vi "setFIFO.vi"(0 "fifoThs":u8, 2 "fifoMode":u8) -> ()   [LabVIEW 2016]
uses:
  #defines.ctl
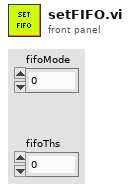
[diagram p1: front panel]
types:
  T1 = typedef "#defines.ctl" = i8
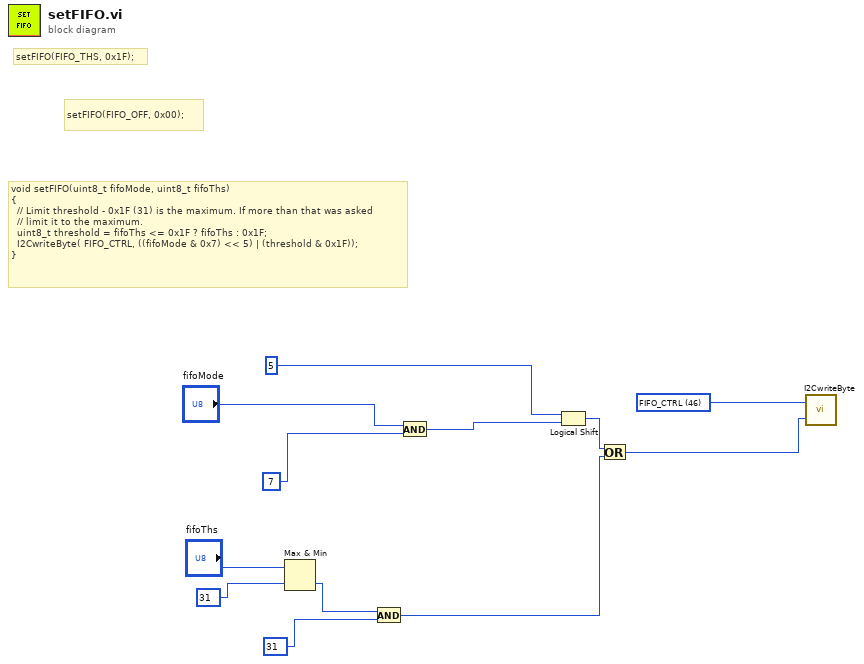
[diagram p0: block diagram]
diagram:
  w8 = T1 46 items=["CTRL_REG9_G"=35, "STATUS_REG_1"=39, "OUT_X_L_XL"=40, "FIFO_CTRL"=46, "FIFO_SRC"=47, "CTRL_REG4_G"=30, "OUT_X_L_G"=24, "OUT_TEMP_L"=21, "INT_GEN_SRC_G"=20, "ORIENT_CFG_G"=19, "CTRL_REG3_G"=18, "CTRL_REG2_G"=17, "CTRL_REG1_G"=16, "WHO_AM_I_XG"=15] ("Ring")
  # "setFIFO(FIFO_OFF, 0x00);"
  # "setFIFO(FIFO_THS, 0x1F);"
  # "void setFIFO(uint8_t fifoMode, uint8_t fifoThs)\n{\n  // Limit threshold - 0x1F (31) is the maximum. If more than that was asked\n  // limit it to the maximum.\n  uint8_t threshold = fifoThs <= 0x1F ? fifoThs : 0x1F;\n  I2CwriteByte( FIFO_CTRL, ((fifoMode & 0x7) << 5) | (threshold & 0x1F));\n}"
  n1 = Max & Min(x="fifoThs", y=u8 31) -> (min(x,y)=w4:u8)  [unwired: 1 out]
  n2 = And(x=w4, y=u8 31) -> (x .and. y?=w1:u8)
  n3 = And(x="fifoMode", y=u8 7) -> (x .and. y?=w11:u8)
  n4 = Logical Shift(y=i16 5, x=w11) -> (x << y=w9:u8)
  n5 = Or(x=w9, y=w1) -> (x .or. y?=w7:u8)
  n6 = call "I2CwriteByte.vi"("data"=w7, "subAddress"=w8) -> ()  [unwired: 1 in]
